vi "test_SessionNeverCreated_CallCloseSessions_CloseNotCalled.vi"(8 "error in":errorcluster) -> (0 "error out":errorcluster, 2 "result":string, 3 "pass":bool)   [LabVIEW 2020, in "MeasurementServerTests.lvlib"]
uses:
  MeasurementServerTests.lvlib
  Runtime/MeasurementLink Session Management/Session Reservation/Session Reservation.lvclass
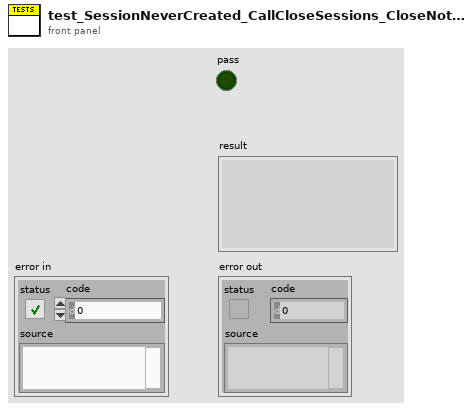
[diagram p1: front panel]
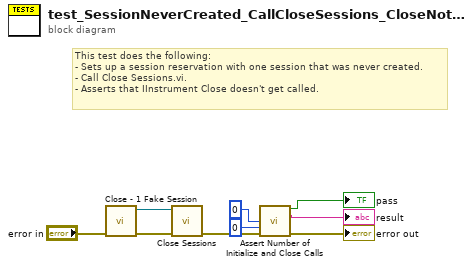
[diagram p0: block diagram]
diagram:
  # "This test does the following:\n- Sets up a session reservation with one session that was never created.\n- Call Close Sessions.vi.\n- Asserts that IInstrument Close doesn't get called."
  n1 = call "Close - 1 Fake Session.vi"("error in (no error)"="error in") -> ("error out"=w8:errorcluster, "Session Reservation out"=w7:refnum<class "Session Reservation.lvclass">)  [unwired: 9 in]
  n2 = call "Close Sessions.vi"("error in"=w8, "session reservation in"=w7) -> ("error out"=w6:errorcluster)  [unwired: 8 in, 1 out]
  n3 = call "Assert Number of Initialize and Close Calls.vi"("expected close-close calls"=u32 0, "expected close-detach calls"=u32 0, "error in"=w6) -> ("pass"=→"pass":bool, "result"=→"result":string, "error out"=→"error out":errorcluster)  [unwired: 10 in]
